vi "raster_scan_ground_shutter_new1.vi"() -> ()   [LabVIEW 2014] (continued)
                        tunnel: w315 -> [w326]
                        i -> [w325]
                        n140 = Quotient & Remainder(x=w325, y=w326) -> (x-y*floor(x/y)=w333:i32)  [unwired: 1 out]
                        n141 = Equal To 0?(x=w333) -> (x = 0?=w332:bool)
                        n142 = case shown="True" w332 {
                          tunnel: w331 -> [w338 w345]
                          tunnel: w330 -> [w339 w343]
                          tunnel: [w339 w342] -> w329
                          tunnel: w328 -> [w337 w341]
                          tunnel: [w335 w341] -> w327
                          tunnel: w325 -> [w334 w340]
                          frame False {
                            # "Raman Pump Off\nOdd Images"
                            n143 = Index Array(array=w338, index (row)=w334) -> (element=w336:dbl[])  [unwired: 1 in]
                            n144 = Add(x=w336, y=w337) -> (x+y=w335:dbl[])
                          }
                          frame True {
                            # "Raman pump on\nEven Images"
                            n145 = Index Array(array=w345, index (row)=w340) -> (element=w344:dbl[])  [unwired: 1 in]
                            n146 = Add(x=w344, y=w343) -> (x+y=w342:dbl[])
                          }
                        }
                      }
                      n147 = Divide(x=w318, y=w316) -> (x/y=w313:dbl[])
                      n148 = Divide(x=w317, y=w316) -> (x/y=w314:dbl[])
                      n149 = Divide(x=w313, y=w314) -> ()  [unwired: 1 out]
                    }
                    frame #2 {
                      # "Calculate the Gain based on the two cursors on the graph"
                      n150 = stacked-sequence {
                        frame #0 {
                          # "Select Cursor 0"
                          n151 = property on="Spectra" class="XYGraph (strict)"("Active Cursor"=0) -> ()  [unwired: 2 in, 2 out]
                        }
                        frame #1 {
                          # "Record the Y position of cursor 0"
                          n152 = property on="Spectra" class="XYGraph (strict)"() -> ("Cursor.Cursor Position:Cursor Y"=→"cursor y":dbl)  [unwired: 2 in, 2 out]
                        }
                        frame #2 {
                          # "Select Cursor 1"
                          n153 = property on="Spectra" class="XYGraph (strict)"("Active Cursor"=1) -> ()  [unwired: 2 in, 2 out]
                        }
                        frame #3 {
                          # "Calculate the Gain"
                          n154 = property on="Spectra" class="XYGraph (strict)"() -> ("Cursor.Cursor Position:Cursor Y"=w349:dbl)  [unwired: 2 in, 2 out]
                          n155 = local read "cursor y"() -> (w354:dbl)
                          n156 = Subtract(x=w349, y=w354) -> (x-y=w351:dbl)
                          n157 = Absolute Value(x=w351) -> (abs(x)=w353:dbl)
                          n158 = Multiply(x=w353, y=100) -> (x*y=→"Gain":dbl)
                        }
                      }
                    }
                    frame #3 {
                      n159 = Wait (ms)(milliseconds to wait=50) -> ()  [unwired: 1 out]
                    }
                  }
                  n160 = call <instrlib>:"_subvi_LivePos_Main.vi"("xCommand"="xCommand", "yCommand"="yCommand", "zCommand"="zCommand", "handle"=w244, "commandZ"="commandZ", "commandY"="commandY", "commandX"="commandX") -> ("xRead"=w255:dbl, "yRead"=w254:dbl, "zRead"=w253:dbl, "counter"=w245:u32)  [unwired: 1 in, 8 out]
                  n161 = Equal To 0?(x=w245) -> (x = 0?=w246:bool)
                  n162 = case shown="True" w246 {
                    tunnel: w255 -> [_ w279]
                    tunnel: w254 -> [_ w278]
                    tunnel: w253 -> [_ w277]
                    frame False {
                    }
                    frame True {
                      "xRead" <- w279
                      "yRead" <- w278
                      "zRead" <- w277
                    }
                  }
                  n163 = local read "Shutter Position"() -> (w242:bool)
                  n164 = local read "Focus"() -> (w243:bool)
                  n165 = local read "Step Size (micro meter)"() -> (w259:dbl)
                  n166 = local read "Start Position"() -> (w270:i32)
                  n167 = local read "MOVE"() -> (w272:bool)
                  n168 = local read "PUMP"() -> (w273:bool)
                  n169 = local read "GO"() -> (w264:bool)
                  n170 = Boolean To (0,1)(Boolean=w273) -> (0, 1=w275:i16)
                  n171 = call "shutter_new.vi"("error in"=w239, "ShutterID"=310, "Shutter Position"=w242, "ObjectPtr"=w240) -> ()  [unwired: 1 out]
                  n172 = Add(x=w275, y=i16 1) -> (x+y=w271:i16)
                  n173 = And(x=w272, y=w276) -> (x .and. y?=w269:bool)
                  n174 = Multiply(x=w259, y=10.0) -> (x*y=w257:dbl)
                  n175 = Round To Nearest(number=w257) -> (nearest integer value=w256:dbl)
                  n176 = call "Pico_move_new.vi"("Motor"=w271, "CmdLib Out"=w268, "DeviceKey Out"=w267, "Start Position"=w270, "Boolean 2"=w264, "Relative Steps"=w256, "Boolean"=w269, "error out"=w265, "Device Address Out"=w266) -> ("CmdLib Out"=w263:refnum<k24>, "DeviceKey Out"=w262:string, "Device Address Out"=w261:i32, "error out 2"=w260:errorcluster)  [unwired: 3 in]
                  n177 = local write "CmdLib Out"(w263) -> ()
                  n178 = local write "Device Address Out"(w261) -> ()
                  n179 = local write "error out 2"(w260) -> ()
                  n180 = local write "DeviceKey Out"(w262) -> ()
                }
              }
            }
          }
          frame #4 {
            n181 = case shown="True" "Ruster Scan" {
              tunnel: w358 -> [_ w402]
              tunnel: w357 -> [_ w376]
              tunnel: w356 -> [_ w375]
              frame False {
                (unwired) FALSE ("Pause 2")
              }
              frame True {
                w394 = dbl[][] []
                # "X Ramp Generator"
                # "Y Ramp Generator"
                n182 = local read "Path"() -> (w362:string)
                n183 = Build Array("X Start  (um)", "X End  (um)", "Y Start  (um)", "Y End  (um)") -> (w393:dbl[])
                n184 = Concatenate Strings(w362, "\\" ("string"), "OFF" ("string")) -> (w364:string)
                n185 = Concatenate Strings("Path", "\\" ("string"), "ON" ("string")) -> (w369:string)
                n186 = Array Max & Min(array=w393) -> (max value=w387:dbl)  [unwired: 3 out]
                n187 = String To Path(string=w364) -> (path=w367:path)
                n188 = String To Path(string=w369) -> (path=w373:path)
                n189 = call "RampGenerator.vi"("Number of Positions"="Y Samples", "End  (um)"="Y End  (um)", "Start  (um)"="Y Start  (um)") -> ("Array"=w396:dbl[])  [unwired: 1 in]
                n190 = Greater?(x=w387, y=70.0) -> (0:w377:bool)
                n191 = call "RampGenerator.vi"("Number of Positions"="X Samples", "End  (um)"="X End  (um)", "Start  (um)"="X Start  (um)") -> ("Array"=w397:dbl[])  [unwired: 1 in]
                n192 = case shown="True" w377 {
                  tunnel: [w404 w406] -> w398
                  tunnel: w396 -> [w404 _]
                  tunnel: [w403 w406] -> w399
                  tunnel: w397 -> [w403 _]
                  frame False {
                  }
                  frame True {
                    w406 = dbl[] [] ("Array")
                    n193 = One Button Dialog(message="Values are \nout of Range") -> ()  [unwired: 1 in, 1 out]
                  }
                }
                n194 = Create Folder(path (use dialog)=w367) -> (created path=w363:path)  [unwired: 2 in, 2 out]
                n195 = Create Folder(path (use dialog)=w373) -> (created path=w368:path)  [unwired: 2 in, 2 out]
                n196 = Path To String(path=w363) -> (string=→"OFF":string)
                n197 = Path To String(path=w368) -> (string=→"ON":string)
                n198 = Array Size(array=w396) -> (size(s)=w395:i32)
                n199 = while {
                  tunnel: w398 -> [w448]
                  tunnel: w402 -> [w447]
                  tunnel: w399 -> [w446]
                  tunnel: "X Start  (um)" -> [w445]
                  shift-right: [w440] -> w378
                  shift-left: w394 -> [w424]
                  shift-right: [w442] -> w382
                  shift-left: w394 -> [w423]
                  tunnel: w377 -> [w414]
                  tunnel: w395 -> [w438]
                  tunnel: "X Start  (um)" -> [w437]
                  tunnel: "X End  (um)" -> [w436]
                  tunnel: "Y Start  (um)" -> [w435]
                  tunnel: "Y End  (um)" -> [w434]
                  shift-right: [w429] -> w383
                  shift-left: w394 -> [w425]
                  shift-right: [w427] -> w386
                  shift-left: w394 -> [w426]
                  tunnel: w376 -> [w412]
                  tunnel: w375 -> [w411]
                  i -> [w444]
                  stop <- w413 stop-if-true
                  n200 = Bundle(w426, w425, w424, w423, w414) -> (w422:T5)  [unwired: 1 in]
                  n201 = Unbundle(w422) -> (w421:dbl[][], w418:dbl[][], w420:dbl[][], w419:dbl[][], w410:bool)
                  n202 = stacked-sequence {
                    seq-local: [w450 _] -> [_ w477]
                    tunnel: w448 -> [w454 _]
                    tunnel: w444 -> [w452 w464]
                    tunnel: w447 -> [w453 w478]
                    tunnel: w446 -> [_ w480]
                    tunnel: w445 -> [_ w479]
                    tunnel: [w451 _] -> w408
                    tunnel: [_ w476] -> w417
                    tunnel: [_ w475] -> w416
                    tunnel: [_ w463] -> w433
                    tunnel: w414 -> [_ w474]
                    tunnel: w410 -> [_ w473]
                    tunnel: w438 -> [_ w472]
                    tunnel: w437 -> [_ w471]
                    tunnel: w436 -> [_ w470]
                    tunnel: w435 -> [_ w469]
                    tunnel: w434 -> [_ w468]
                    tunnel: [_ w466] -> w415
                    tunnel: [_ w465] -> w432
                    tunnel: w412 -> [_ w462]
                    tunnel: w411 -> [_ w461]
                    tunnel: [_ w460] -> w407
                    frame #0 {
                      w457 = 2  # Y AXIS
                      # "Step the Y axis"
                      n203 = Array Size(array=w454) -> (size(s)=w449:i32)
                      n204 = Index Array(array=w454, index=w452) -> (element=w455:dbl)
                      n205 = Increment(x=w452) -> (x+1=w456:i32)
                      n206 = Subtract(x=w449, y=w456) -> (x-y=w459:i32)
                      n207 = Equal To 0?(x=w459) -> (x = 0?=w451:bool)
                      n208 = call "WriteReadN.vi"("Handle"=w453, "Axis"=w457, "Delay (ms)"="Y Delay (ms)", "Move to (um)"=w455) -> ("Current Position (um)"=w450:dbl)
                      "Y Position (um)" <- w450
                    }
                    frame #1 {
                      w467 = dbl[] []
                      n209 = while {
                        tunnel: w480 -> [w514]
                        tunnel: w479 -> [w513]
                        tunnel: w478 -> [w511]
                        tunnel: w477 -> [w510]
                        tunnel: w464 -> [w497]
                        shift-right: [w509] -> w476
                        shift-left: w467 -> [w496]
                        shift-right: [w508] -> w475
                        shift-left: w467 -> [w495]
                        tunnel: w474 -> [w507]
                        tunnel: w473 -> [w505]
                        tunnel: w472 -> [w504]
                        tunnel: w471 -> [w503]
                        tunnel: w470 -> [w502]
                        tunnel: w469 -> [w501]
                        tunnel: w468 -> [w500]
                        shift-right: [w499] -> w466
                        shift-left: w467 -> [w494]
                        shift-right: [w498] -> w465
                        shift-left: w467 -> [w490]
                        tunnel: w464 -> [w487]
                        tunnel: [w486] -> w463
                        tunnel: w462 -> [w485]
                        tunnel: w461 -> [w484]
                        tunnel: [w481] -> w460
                        i -> [w512]
                        stop <- w506 stop-if-true
                        n210 = Bundle(w496, w495, w490, w494, w487) -> (w493:cluster{dbl[], dbl[], dbl[], dbl[], i32})  [unwired: 1 in]
                        n211 = Unbundle(w493) -> (w492:dbl[], w491:dbl[], w489:dbl[], w488:dbl[], w486:i32)
                        n212 = stacked-sequence {
                          seq-local: [w532 _] -> [_ w572]
                          tunnel: w514 -> [w537 _]
                          tunnel: w513 -> [_ _]
                          tunnel: w512 -> [w528 _]
                          tunnel: w511 -> [w545 _]
                          tunnel: [w544 _] -> w483
                          tunnel: w510 -> [w543 w573]
                          tunnel: w497 -> [w530 _]
                          tunnel: w492 -> [_ w564]
                          tunnel: [_ w563] -> w509
                          tunnel: [_ w557] -> w508
                          tunnel: w491 -> [_ w566]
                          tunnel: w507 -> [_ _]
                          tunnel: w504 -> [w531 _]
                          tunnel: w503 -> [w520 _]
                          tunnel: w502 -> [w519 _]
                          tunnel: w501 -> [w517 _]
                          tunnel: w500 -> [w518 _]
                          tunnel: w488 -> [_ w561]
                          tunnel: [_ w560] -> w499
                          tunnel: w489 -> [_ w569]
                          tunnel: [_ w567] -> w498
                          tunnel: w485 -> [_ w556]
                          tunnel: w484 -> [_ w555]
                          tunnel: [_ w554] -> w481
                          frame #0 {
                            w546 = 1  # X AXIS
                            # "Step the X axis"
                            n213 = Quotient & Remainder(x=w530, y=2) -> (x-y*floor(x/y)=w541:i32)  [unwired: 1 out]
                            n214 = Array Size(array=w537) -> (size(s)=w529:i32)
                            n215 = Equal?(x=w541, y=0) -> (x = y?=w534:bool)
                            n216 = Multiply(x=w529, y=w530) -> (x*y=w526:i32)
                            n217 = Increment(x=w528) -> (x+1=w527:i32)
                            n218 = Subtract(x=w529, y=1) -> (x-y=w535:i32)
                            n219 = Add(x=w526, y=w527) -> (x+y=w523:i32)
                            n220 = Multiply(x=w531, y=w529) -> (x*y=w522:i32)
                            n221 = Divide(x=w523, y=w522) -> (x/y=w525:dbl)
                            n222 = Subtract(x=w535, y=w528) -> (x-y=w538:i32)
                            n223 = case shown="False" w534 {
                              tunnel: w537 -> [w549 w553]
                              tunnel: w528 -> [_ w552]
                              tunnel: [w550 w551] -> w539
                              tunnel: w538 -> [w548 _]
                              frame False {
                                n224 = Index Array(array=w549, index=w548) -> (element=w550:dbl)
                              }
                              frame True {
                                n225 = Index Array(array=w553, index=w552) -> (element=w551:dbl)
                              }
                            }
                            n226 = Multiply(x=w525, y=100.0) -> (x*y=→"Progress (%)":dbl)
                            n227 = Equal To 0?(x=w538) -> (x = 0?=w544:bool)
                            n228 = Not Equal?(x=w522, y=w523) -> (x != y?=w516:bool)
                            "?" <- w516
                            n229 = call "WriteReadN.vi"("Handle"=w545, "Axis"=w546, "Delay (ms)"="X Deyal (ms)", "Move to (um)"=w539) -> ("Current Position (um)"=w532:dbl)
                            "X Position (um)" <- w532
                            n230 = Not(x=w516) -> (.not. x?=w521:bool)
                            n231 = call "?"("Reset"=w521, "Y Input"=w543, "X Input"=w532) -> ("XY Graph"=→"XY Graph":cluster{"X":dbl[], "Y":dbl[]}[])  [unwired: 7 in, 1 out]
                            n232 = property on="XY Graph" class="XYGraph (strict)"("XScale.Maximum"=w519) -> ()  [unwired: 2 in, 2 out]
                            n233 = property on="XY Graph" class="XYGraph (strict)"("YScale.Minimum"=w517) -> ()  [unwired: 2 in, 2 out]
                            n234 = property on="XY Graph" class="XYGraph (strict)"("YScale.Maximum"=w518) -> ()  [unwired: 2 in, 2 out]
                            n235 = property on="XY Graph" class="XYGraph (strict)"("XScale.Minimum"=w520) -> ()  [unwired: 2 in, 2 out]
                          }
                          frame #1 {
                            w570 = 0.0
                            w571 = 0.0
                            n236 = for {
                              N: "Sets" -> [w593]
                              tunnel: w572 -> [w603]
                              tunnel: w573 -> [w602]
                              shift-right: [w600] -> w562
                              shift-left: w571 -> [w588]
                              shift-right: [w599] -> w565
                              shift-left: w570 -> [w587]
                              shift-right: [w595] -> w568
                              shift-left: w571 -> [w589]
                              shift-right: [w594] -> w558
                              shift-left: w570 -> [w590]
                              tunnel: w556 -> [w580]
                              tunnel: w555 -> [w579]
                              tunnel: [w575] -> w554
                              i -> [w604]
                              n237 = Increment(x=w604) -> (x+1=w581:i32)
                              "Current Set" <- w581
                              n238 = local read item#69() -> (w591:bool)
                              n239 = Bundle(w590, w589, w588, w587) -> (w586:cluster{dbl, dbl, dbl, dbl})  [unwired: 1 in]
                              n240 = Not Equal?(x=w593, y=w581) -> (x != y?=w592:bool)
                              n241 = Not Or(1:w591, 2:w592) -> (0:w577:bool)
                              n242 = Not(x=w577) -> (.not. x?=w576:bool)
                              n243 = stacked-sequence {
                                tunnel: w581 -> [w605 _ _]
                                tunnel: w603 -> [w613 _ _]
                                tunnel: w602 -> [w612 _ _]
                                tunnel: [w611 _ _] -> w601
                                tunnel: [w610 _ _] -> w598
                                tunnel: [w609 _ _] -> w597
                                tunnel: [w608 _ _] -> w596
                                tunnel: w580 -> [w607 _ _]
                                tunnel: w579 -> [w606 _ _]
                                tunnel: [_ _ "STOP Scan"] -> w575
                                frame #0 {
                                n244 = stacked-sequence {
                                seq-local: [_ "# Images" _ _ _ _ _ _] -> [_ _ _ _ _ w698 _ _]
                                seq-local: [_ w622 _ _ _ _ _ _] -> [_ _ w650 _ _ _ w719 _]
                                tunnel: w613 -> [_ _ _ w673 _ _ _ w740]
                                tunnel: w612 -> [_ _ _ w672 _ _ _ w739]
                                tunnel: [_ _ w652 _ _ _ _ _] -> w611
                                tunnel: [_ _ w651 _ _ _ _ _] -> w610
                                tunnel: w605 -> [_ _ _ w674 _ _ _ w741]
                                tunnel: [_ _ _ _ _ _ w718 _] -> w609
                                tunnel: [_ _ _ _ _ _ w717 _] -> w608
                                tunnel: w607 -> [w615 _ _ _ w682 _ _ _]
                                tunnel: w606 -> [w614 _ _ _ w681 _ _ _]
                                frame #0 {
                                n245 = flat-sequence {
                                tunnel: w615 -> [w619]
                                tunnel: w614 -> [w618]
                                frame #0 {
                                n246 = call "shutter_new.vi"("error in"=w618, "ShutterID"=310, "Shutter Position"=TRUE, "ObjectPtr"=w619) -> ()  [unwired: 1 out]
                                }
                                frame #1 {
                                n247 = Wait (ms)(milliseconds to wait=u32 200) -> ()  [unwired: 1 out]
                                }
                                }
                                }
                                frame #1 {
                                n248 = local read "Camera Handle"() -> (w639:u32)
                                n249 = local read "error out"() -> (w638:errorcluster)
                                n250 = call "DataGrabber.vi"("# Images In"="# Images", "Camera Handle"=w639, "error in (no error)"=w638) -> ("# Images Out"=w632:u16, "Camera Handle"=w636:u32, "Data"=w635:dbl[][], "error out"=w637:errorcluster)
                                n251 = case shown="True" "Change to Raman Shift" {
                                tunnel: [w641 w643] -> w622
                                tunnel: ["Pixel" ("X Scale.Name Label.Text") "Raman Shift (cm-1)" ("X Scale.Name Label.Text")] -> w625
                                frame False {
                                n252 = local read "Result"() -> (w641:dbl[])
                                }
                                frame True {
                                n253 = local read "Result 2"() -> (w643:dbl[])
                                }
                                }
                                n254 = local write "Camera Handle"(w636) -> ()
                                n255 = local write "error out"(w637) -> ()
                                n256 = local write "# Images"(w632) -> ()
                                n257 = local read "Bkgndoff"() -> (w633:dbl[])
                                n258 = local read "Bkgndon"() -> (w634:dbl[])
                                n259 = call "DataProcessor.vi"("PumpOffBkgd"=w633, "PumpOnBkgd"=w634, "Data"=w635, "# of Images"=w632) -> ("PumpOff"=w621:dbl[], "PumpOn"=w630:dbl[], "Raman"=w629:dbl[])
                                "Ground" <- w629
                                "On" <- w630
                                "Off" <- w621
                                "Raman" <- w629
                                n260 = local read "Flip Spectra"() -> (w624:bool)
                                n261 = local write "Waveform Graph"(w621) -> ()
                                n262 = property on="Spectra" class="XYGraph (strict)"("XScale.NameLbl.Text"=w625) -> ()  [unwired: 2 in, 2 out]
                                n263 = local write "On"(w630) -> ()
                                n264 = local write "Off"(w621) -> ()
                                n265 = Not(x=w624) -> (.not. x?=w623:bool)
                                n266 = case shown="True" w623 {
                                tunnel: w629 -> [w644 w646]
                                tunnel: [w645 w646] -> w628
                                frame False {
                                n267 = Reciprocal(x=w644) -> (1/x=w645:dbl[])
                                }
                                frame True {
                                }
                                }
                                n268 = Build Cluster Array(w622, w628) -> (→"Spectra":cluster{dbl, dbl}[])
                                }
                                frame #2 {
                                # "Peak fitting and intergation"
                                n269 = local read "Raman"() -> (w653:dbl[])
                                n270 = property on="Spectra" class="XYGraph (strict)"("Active Cursor"=u32 1) -> ("Cursor.Cursor X"=w655:dbl)  [unwired: 2 in, 2 out]
                                n271 = property on="Spectra" class="XYGraph (strict)"("Active Cursor"=u32 0) -> ("Cursor.Cursor X"=w656:dbl)  [unwired: 2 in, 2 out]
                                n272 = call "fit_new.vi"("Filter ?"="Filter?", "parameter bounds"="parameter bounds", "Cursor1 2"=w655, "Cursor1"=w656, "array 2"=w650, "array"=w653, "Enum"="Enum", "Initial Parameters"="Initial Parameters") -> ("Intergrate"=w651:dbl, "Fit"=w652:dbl)  [unwired: 2 in]
                                "FIT" <- w652
                                "AREA" <- w651
                                }
                                frame #3 {
                                # "Here we save spectrum for each special point"
                                n273 = local read "ON"() -> (w667:string)
                                n274 = Format Into String(w674) -> (resulting string=w660:string)  [unwired: 3 in, 1 out]
                                n275 = call "number_to_sring.vi"("Numeric"=w673) -> ("result string"=w665:string)  [unwired: 10 in]
                                n276 = call "number_to_sring.vi"("Numeric"=w672) -> ("result string"=w663:string)  [unwired: 10 in]
                                n277 = Concatenate Strings(w667, "\\", "Filename", "_", "X_" ("string"), w665, "_Y_" ("string"), w663, "_ON" ("string"), "_" ("string"), w660) -> (w671:string)
                                "File_name" <- w671
                                n278 = local read "Ground"() -> (w659:dbl[])
                                n279 = local read "On"() -> (w680:dbl[])
                                n280 = local read "Off"() -> (w679:dbl[])
                                n281 = String To Path(string=w671) -> (path=w677:path)
                                n282 = Build Array(w659, w680, w679) -> (w678:dbl[][])
                                n283 = call-poly <vilib>:"Write To Spreadsheet File.vi"("transpose? (no:F)"=TRUE, "format (%.3f)"="%.7f", "2D data"=w678, "file path (dialog if empty)"=w677) -> ()  [unwired: 4 in, 1 out]
                                }
                                frame #4 {
                                n284 = flat-sequence {
                                tunnel: w682 -> [w686]
                                tunnel: w681 -> [w685]
                                frame #0 {
                                n285 = call "shutter_new.vi"("error in"=w685, "ShutterID"=310, "Shutter Position"=FALSE, "ObjectPtr"=w686) -> ()  [unwired: 1 out]
                                }
                                frame #1 {
                                n286 = Wait (ms)(milliseconds to wait=u32 200) -> ()  [unwired: 1 out]
                                }
                                }
                                }
                                frame #5 {
                                n287 = local read "Camera Handle"() -> (w706:u32)
                                n288 = local read "error out"() -> (w705:errorcluster)
                                n289 = local read "Change to Raman Shift"() -> (w694:bool)
                                n290 = call "DataGrabber.vi"("# Images In"=w698, "Camera Handle"=w706, "error in (no error)"=w705) -> ("# Images Out"=w699:u16, "Camera Handle"=w703:u32, "Data"=w702:dbl[][], "error out"=w704:errorcluster)
                                n291 = local write "Camera Handle"(w703) -> ()
                                n292 = local write "error out"(w704) -> ()
                                n293 = local write "# Images"(w699) -> ()
                                n294 = local read "Bkgndoff"() -> (w700:dbl[])
                                n295 = local read "Bkgndon"() -> (w701:dbl[])
                                n296 = case shown="False" w694 {
                                tunnel: [w708 w710] -> w693
                                tunnel: ["Pixel" ("X Scale.Name Label.Text") "Raman Shift (cm-1)" ("X Scale.Name Label.Text")] -> w695
                                frame False {
                                n297 = local read "Result"() -> (w708:dbl[])
                                }
                                frame True {
                                n298 = local read "Result 2"() -> (w710:dbl[])
                                }
                                }
                                n299 = call "DataProcessor.vi"("PumpOffBkgd"=w700, "PumpOnBkgd"=w701, "Data"=w702, "# of Images"=w699) -> ("PumpOff"=w688:dbl[], "PumpOn"=w697:dbl[], "Raman"=w696:dbl[])
                                n300 = local read "Flip Spectra"() -> (w690:bool)
                                n301 = local write "Waveform Graph"(w688) -> ()
                                n302 = Not(x=w690) -> (.not. x?=w689:bool)
                                n303 = local write "On"(w697) -> ()
                                n304 = local write "Off"(w688) -> ()
                                n305 = case shown="True" w689 {
                                tunnel: w696 -> [w712 w713]
                                tunnel: [w711 w713] -> w692
                                frame False {
                                n306 = Reciprocal(x=w712) -> (1/x=w711:dbl[])
                                }
                                frame True {
                                }
                                }
                                n307 = property on="Spectra" class="XYGraph (strict)"("XScale.NameLbl.Text"=w695) -> ()  [unwired: 2 in, 2 out]
                                n308 = local write "Ground"(w696) -> ()
                                n309 = local write "Raman"(w696) -> ()
                                n310 = Build Cluster Array(w693, w692) -> (w691:cluster{dbl, dbl}[])
                                n311 = local write "Off"(w688) -> ()
                                n312 = local write "Spectra"(w691) -> ()
                                n313 = local write "On"(w697) -> ()
                                }
                                frame #6 {
                                # "Peak fitting and intergation"
                                n314 = local read "Raman"() -> (w720:dbl[])
                                n315 = local read "Initial Parameters"() -> (w721:T2)
                                n316 = local read "Enum"() -> (w716:enum16{"Lorantzian", "fano", "gaussian"})
                                n317 = property on="Spectra" class="XYGraph (strict)"("Active Cursor"=u32 0) -> ("Cursor.Cursor X"=w723:dbl)  [unwired: 2 in, 2 out]
                                n318 = property on="Spectra" class="XYGraph (strict)"("Active Cursor"=u32 1) -> ("Cursor.Cursor X"=w722:dbl)  [unwired: 2 in, 2 out]
                                n319 = local read "Filter?"() -> (w714:bool)
                                n320 = local read "parameter bounds"() -> (w715:T1)
                                n321 = call "fit_new.vi"("Filter ?"=w714, "parameter bounds"=w715, "Cursor1 2"=w722, "Cursor1"=w723, "array 2"=w719, "array"=w720, "Enum"=w716, "Initial Parameters"=w721) -> ("Intergrate"=w717:dbl, "Fit"=w718:dbl)  [unwired: 2 in]
                                n322 = local write "AREA"(w717) -> ()
                                n323 = local write "FIT"(w718) -> ()
                                }
                                frame #7 {
                                # "Here we save spectrum for each special point"
                                n324 = local read "Filename"() -> (w736:string)
                                n325 = Format Into String(w741) -> (resulting string=w727:string)  [unwired: 3 in, 1 out]
                                n326 = call "number_to_sring.vi"("Numeric"=w740) -> ("result string"=w732:string)  [unwired: 10 in]
                                n327 = local read "OFF"() -> (w734:string)
                                n328 = call "number_to_sring.vi"("Numeric"=w739) -> ("result string"=w730:string)  [unwired: 10 in]
                                n329 = Concatenate Strings(w734, "\\", w736, "_", "X_" ("string"), w732, "_Y_" ("string"), w730, "_OFF" ("string"), "_" ("string"), w727) -> (w738:string)
                                n330 = local read "Ground"() -> (w726:dbl[])
                                n331 = local read "Off"() -> (w747:dbl[])
                                n332 = local read "Off"() -> (w746:dbl[])
                                n333 = String To Path(string=w738) -> (path=w744:path)
                                n334 = local write "File_name"(w738) -> ()
                                n335 = Build Array(w726, w747, w746) -> (w745:dbl[][])
                                n336 = call-poly <vilib>:"Write To Spreadsheet File.vi"("transpose? (no:F)"=TRUE, "format (%.3f)"="%.7f", "2D data"=w745, "file path (dialog if empty)"=w744) -> ()  [unwired: 4 in, 1 out]
                                }
                                }
                                }
                                frame #1 {
                                n337 = stacked-sequence {
                                frame #0 {
                                n338 = property on="Spectra" class="XYGraph (strict)"("Active Cursor"=0) -> ()  [unwired: 2 in, 2 out]
                                }
                                frame #1 {
                                n339 = property on="Spectra" class="XYGraph (strict)"() -> ("Cursor.Cursor Position:Cursor Y"=w749:dbl)  [unwired: 2 in, 2 out]
                                n340 = local write "cursor y"(w749) -> ()
                                }
                                frame #2 {
                                n341 = property on="Spectra" class="XYGraph (strict)"("Active Cursor"=1) -> ()  [unwired: 2 in, 2 out]
                                }
                                frame #3 {
                                n342 = property on="Spectra" class="XYGraph (strict)"() -> ("Cursor.Cursor Position:Cursor Y"=w751:dbl)  [unwired: 2 in, 2 out]
                                n343 = local read "cursor y"() -> (w752:dbl)
                                n344 = Subtract(x=w751, y=w752) -> (x-y=w754:dbl)
                                n345 = Absolute Value(x=w754) -> (abs(x)=w756:dbl)
                                n346 = Multiply(x=w756, y=100) -> (x*y=w753:dbl)
                                n347 = local write "Gain"(w753) -> ()
                                }
                                }
                                }
                                frame #2 {
                                n348 = while {
                                stop <- "Pause" continue-if-true
                                }
                                }
                              }
                              n349 = Not(x=w575) -> (.not. x?=w574:bool)
                              n350 = And(x=w576, y=w574) -> (x .and. y?=→"Scanig":bool)
                              n351 = Unbundle(w586) -> (w585:dbl, w584:dbl, w583:dbl, w582:dbl)
                              n352 = Add(x=w598, y=w582) -> (x+y=w599:dbl)
                              n353 = Add(x=w596, y=w585) -> (x+y=w594:dbl)
                              n354 = Add(x=w601, y=w583) -> (x+y=w600:dbl)
                              n355 = Add(x=w597, y=w584) -> (x+y=w595:dbl)
                            }
                            n356 = call "array.vi"("x"=w558, "y"="Sets", "array"=w561) -> ("appended array"=w560:dbl[])  [unwired: 6 in]
                            n357 = call "array.vi"("x"=w562, "y"="Sets", "array"=w564) -> ("appended array"=w563:dbl[])  [unwired: 6 in]
                            n358 = call "array.vi"("x"=w565, "y"="Sets", "array"=w566) -> ("appended array"=w557:dbl[])  [unwired: 6 in]
                            n359 = call "array.vi"("x"=w568, "y"="Sets", "array"=w569) -> ("appended array"=w567:dbl[])  [unwired: 6 in]
                          }
                        }
                        n360 = Or(x=w483, y=w481) -> (x .or. y?=w482:bool)
                        n361 = Or(x=w505, y=w482) -> (x .or. y?=w506:bool)
                      }
                    }
                  }
                  n362 = Or(x=w408, y=w407) -> (x .or. y?=w409:bool)
                  n363 = Or(x=w410, y=w409) -> (x .or. y?=w413:bool)
                  n364 = call "rotate.vi"("Array in"=w432, "i"=w433) -> ("Array out"=w430:dbl[])  [unwired: 9 in]
                  n365 = call "rotate.vi"("Array in"=w415, "i"=w433) -> ("Array out"=w431:dbl[])  [unwired: 9 in]
                  n366 = call "rotate.vi"("Array in"=w416, "i"=w433) -> ("Array out"=w443:dbl[])  [unwired: 9 in]
                  n367 = call "rotate.vi"("Array in"=w417, "i"=w433) -> ("Array out"=w441:dbl[])  [unwired: 9 in]
                  n368 = Build Array (concatenate)(w430, w421) -> (w427:dbl[][])
                  n369 = Transpose 2D Array(2D array=w427) -> (transposed array=→"DCP OFF":dbl[][])
                  n370 = Build Array (concatenate)(w431, w418) -> (w429:dbl[][])
                  n371 = Build Array (concatenate)(w441, w420) -> (w440:dbl[][])
                  n372 = Transpose 2D Array(2D array=w440) -> (transposed array=→"DCP ON":dbl[][])
                  n373 = Build Array (concatenate)(w443, w419) -> (w442:dbl[][])
                }
                n374 = local read "Filename"() -> (w374:string)
                n375 = local read "Path"() -> (w379:string)
                n376 = call "save_file.vi"("string 3"="_area_ON" ("string"), "string 2"=w374, "string"=w379, "2D data"=w382) -> ()  [unwired: 8 in]
                n377 = call "save_file.vi"("string 3"="_fit_ON" ("string"), "string 2"=w374, "string"=w379, "2D data"=w378) -> ()  [unwired: 8 in]
                n378 = call "save_file.vi"("string 3"="_area_OFF" ("string"), "string 2"=w374, "string"=w379, "2D data"=w383) -> ()  [unwired: 8 in]
                n379 = call "save_file.vi"("string 3"="_fit_OFF" ("string"), "string 2"=w374, "string"=w379, "2D data"=w386) -> ()  [unwired: 8 in]
              }
            }
          }
          frame #5 {
            n380 = case shown="True" "Save" {
              frame False {
              }
              frame True {
                n381 = local read "Raman"() -> (w782:dbl[])
                n382 = local read "Off"() -> (w780:dbl[])
                n383 = local read "On"() -> (w781:dbl[])
                n384 = local read "Path"() -> (w779:string)
                n385 = Build Array(w782, w781, w780) -> (w773:dbl[][])
                n386 = local read "Filename"() -> (w777:string)
                n387 = Concatenate Strings(w779, "\\", w777) -> (w776:string)
                n388 = String To Path(string=w776) -> (path=w772:path)
                n389 = call-poly <vilib>:"Write To Spreadsheet File.vi"("transpose? (no:F)"=TRUE, "format (%.3f)"="%.7f", "2D data"=w773, "file path (dialog if empty)"=w772) -> ()  [unwired: 4 in, 1 out]
              }
            }
            n390 = case shown="True" "subtract" {
              frame False {
              }
              frame True {
                n391 = local read "Change to Raman Shift"() -> (w790:bool)
                n392 = local read "Subtrarray"() -> (w794:dbl[])
                n393 = local read "Raman"() -> (w793:dbl[])
                n394 = Multiply(x="Scale factor", y=w794) -> (x*y=w792:dbl[])
                n395 = Subtract(x=w793, y=w792) -> (x-y=w788:dbl[])
                n396 = case shown="True" w790 {
                  tunnel: [w797 w799] -> w789
                  tunnel: ["Pixel" ("X Scale.Name Label.Text") "Raman Shift (cm-1)" ("X Scale.Name Label.Text")] -> w791
                  frame False {
                    n397 = local read "Result"() -> (w797:dbl[])
                  }
                  frame True {
                    n398 = local read "Result 2"() -> (w799:dbl[])
                  }
                }
                n399 = property on="Spectra" class="XYGraph (strict)"("XScale.NameLbl.Text"=w791) -> ()  [unwired: 2 in, 2 out]
                n400 = Build Cluster Array(w789, w788) -> (w787:cluster{dbl, dbl}[])
                n401 = local write "Spectra"(w787) -> ()
              }
            }
            n402 = case shown="True" "ChooseBkgdFile" {
              frame False {
              }
              frame True {
                n403 = call-poly <vilib>:"Read From Spreadsheet File.vi"("transpose (no:F)"=TRUE) -> ("first row"=w801:dbl[], "new file path (Not A Path if cancelled)"=→"Background File":path)  [unwired: 6 in, 3 out]
                n404 = Array Subset(array=w801, index=0, length=1340) -> (→"Subtrarray":dbl[])
              }
            }
            n405 = case shown="True" "SetPath" {
              frame False {
              }
              frame True {
                (unwired) 5
                n406 = File Dialog(11:path "C:/DATA") -> (0:w783:errorcluster, 3:w786:path)  [unwired: 6 in, 2 out]
                n407 = Unbundle(w783) -> ()  [unwired: 3 out]
                n408 = Path To String(path=w786) -> (string=w784:string)
                n409 = local write "Path"(w784) -> ()
              }
            }
            n410 = case shown="True" "Boolean" {
              frame False {
              }
              frame True {
                n411 = local read "Path"() -> (w768:string)
                n412 = local read "Filename"() -> (w770:string)
                n413 = Concatenate Strings(w768, "\\", w770) -> (w771:string)
                n414 = String To Path(string=w771) -> (path=w767:path)
                n415 = local read "Off"() -> (w764:dbl[])
                n416 = call-poly <vilib>:"Write To Spreadsheet File.vi"("transpose? (no:F)"=TRUE, "format (%.3f)"="%.7f", "1D data"=w764, "file path (dialog if empty)"=w767) -> ()  [unwired: 4 in, 1 out]
              }
            }
          }
          frame #6 {
            n417 = case shown="True" "Time" {
              frame False {
              }
              frame True {
                n418 = while {
                  shift-right: [w808] -> _
                  shift-left: _ -> [w807]
                  i -> [w809]
                  stop <- "?" stop-if-true
                  n419 = stacked-sequence {
                    seq-local: [w811 _ _] -> [_ _ w857]
                    tunnel: w809 -> [_ w838 _]
                    tunnel: [_ _ w854] -> w808
                    tunnel: w807 -> [_ _ w853]
                    frame #0 {
                      n420 = local read "Change to Raman Shift"() -> (w813:bool)
                      n421 = local read "# Images"() -> (w812:u16)
                      n422 = local read "Camera Handle"() -> (w829:u32)
                      n423 = local read "error out"() -> (w828:errorcluster)
                      n424 = call "DataGrabber.vi"("# Images In"=w812, "Camera Handle"=w829, "error in (no error)"=w828) -> ("# Images Out"=w822:u16, "Camera Handle"=w826:u32, "Data"=w825:dbl[][], "error out"=w827:errorcluster)
                      n425 = local write "Camera Handle"(w826) -> ()
                      n426 = local write "error out"(w827) -> ()
                      n427 = case shown="False" w813 {
                        tunnel: [w831 w833] -> w811
                        tunnel: ["Pixel" ("X Scale.Name Label.Text") "Raman Shift (cm-1)" ("X Scale.Name Label.Text")] -> w815
                        frame False {
                          n428 = local read "Result"() -> (w831:dbl[])
                        }
                        frame True {
                          n429 = local read "Result 2"() -> (w833:dbl[])
                        }
                      }
                      n430 = local write "# Images"(w822) -> ()
                      n431 = local read "Bkgndoff"() -> (w823:dbl[])
                      n432 = local read "Bkgndoff"() -> (w824:dbl[])
                      n433 = call "DataProcessor.vi"("PumpOffBkgd"=w823, "PumpOnBkgd"=w824, "Data"=w825, "# of Images"=w822) -> ("PumpOff"=w821:dbl[], "PumpOn"=w820:dbl[], "Raman"=w814:dbl[])
                      n434 = local read "Flip Spectra"() -> (w817:bool)
